vi "Write Meta Data (UDP Ref).vi"(4 "address":cluster{"address":u32, "port":u16}, 6 "options":T1={"ignore timeout error"=TRUE, "timeout ms (1000)"=1000}, 7 "meta data":T3[](array[typedef]), 8 "error in":errorcluster, 11 "connection ID":refnum<k16>) -> (0 "error out":errorcluster, 3 "connection info out":T2)   [LabVIEW 2010, in "NI STM.lvlib"]
doc: "Use this VI to transmit the meta data cluster to a remote computer. Sending the meta data to another computer helps maintainability since the data resides only on one side and it is shared to other computers at run time."
uses:
  NI STM.lvlib
  SubVIs/MetaDataElement.ctl
  UDP Connection Info.ctl
  UDP Write Options.ctl
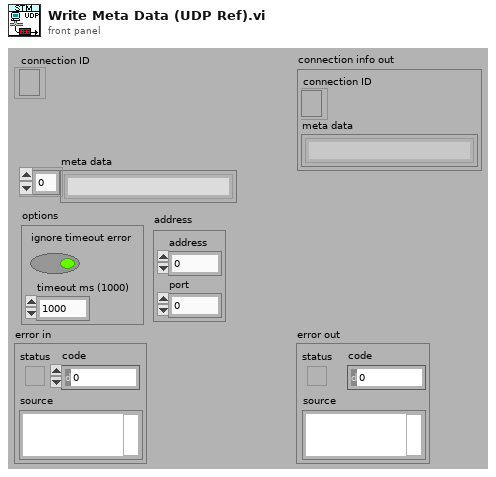
[diagram p1: front panel]
types:
  T1 = typedef "NI STM.lvlib/UDP Write Options.ctl" = cluster{"ignore timeout error":bool, "timeout ms (1000)":i32}
  T2 = typedef "NI STM.lvlib/UDP Connection Info.ctl" = cluster{"connection ID":refnum<k16>, "meta data":T3[]}
  T3 = typedef "NI STM.lvlib/MetaDataElement.ctl" = string
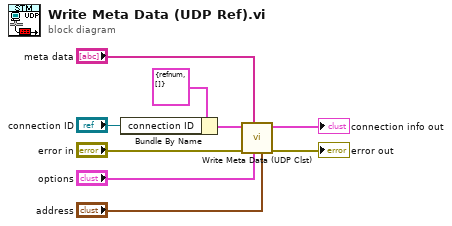
[diagram p0: block diagram]
diagram:
  n1 = Bundle By Name(cluster=T2 {"connection ID"=refnum, "meta data"=[]} ("Connection Info Out"), "connection ID"="connection ID") -> (w7:T2)
  n2 = call "Write Meta Data (UDP Clst).vi"("address"="address", "options"="options", "meta data"="meta data", "error in"="error in", "connection info in"=w7) -> ("error out"=→"error out":errorcluster, "connection info out"=→"connection info out":T2)  [unwired: 5 in]
